vi "decodex_21.vi"() -> ()   [LabVIEW 2021]
doc: "This is a Decodex v2.1\n\nAndré Romero - 2026\nandretec@ifsc.usp.br\nIFSC - USP"
uses:
  <vilib>/Analysis/baseanly.llb/Mean (DBL).vi
  Thorlabs-Vector-Move/aptTec/Thorlabs-V2/Global Motors.vi
  <vilib>/Analysis/NI_AALBase.lvlib
panel:
  out "Layer":dbl[][](array[numeric])
  out "Motor Y":bool=TRUE
  out "Motor X":bool=TRUE
  out "Motor Z":bool=TRUE
  out "Estimated final time":string
  out "Total Estimated Time":string
  out "Total Layer Time":string
  in  "Dynamic/Manual":bool=TRUE
  in  "Mult factor":dbl=1.0
  out "Current velocity (m/s)":dbl=100.0
  out "End time":string
  out "Start time":string="5:55 PM"
  out "Total Time":string
  in  "Stop Button":bool
  out "Total Lines":i32=41
  out "Total Layers":i32=27
  out "Z initial":dbl=0.020260028541088104 format="%#_2g"
  in  "Z on/off":bool=TRUE
  in  "Layer height (mm)":dbl=1.0
  in  "file path (use dialog)":path=path "C:/user-Lab/AndreTec/SolidWorks/cubo_3_LH_06um_LW_06um_lines_3_XYSV.txt"
  out "Layer":i32=1
  out "Line":i32
  in  "Velocity (m/s)":dbl=30.0
  in  "X":refnum<k7>(container)
  in  "Y":refnum<k7>(container)
  in  "Z":refnum<k7>(container)
  # "mm"
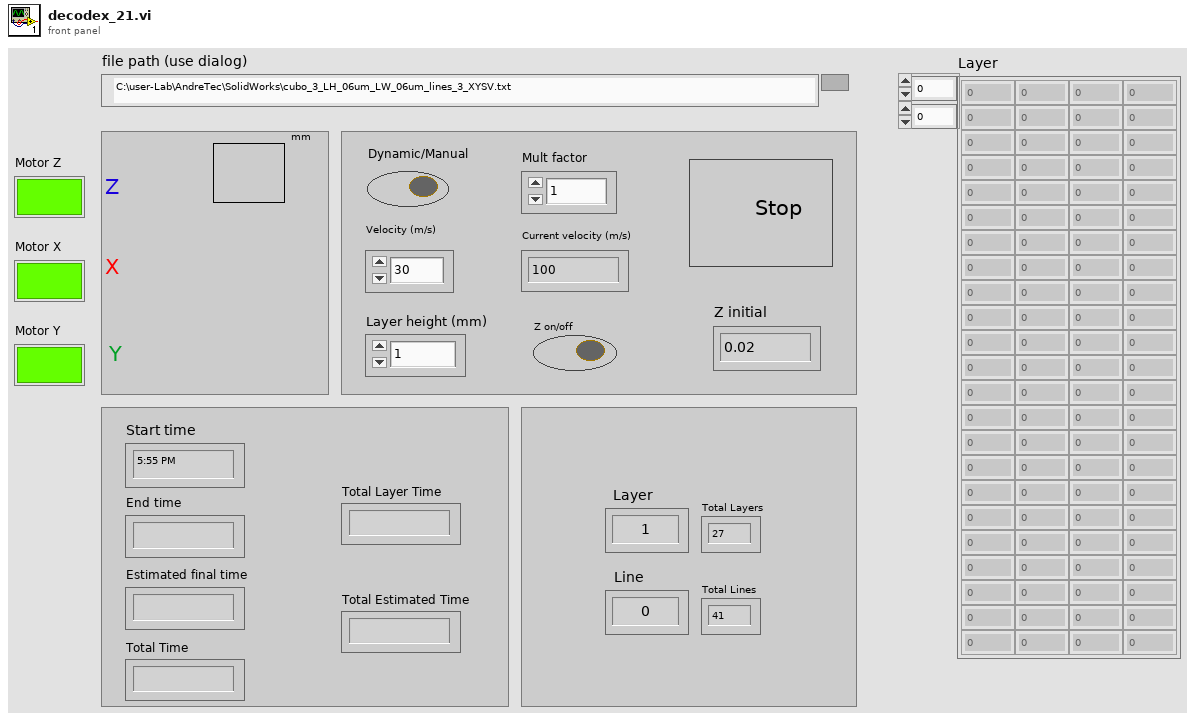
[diagram p1: front panel]
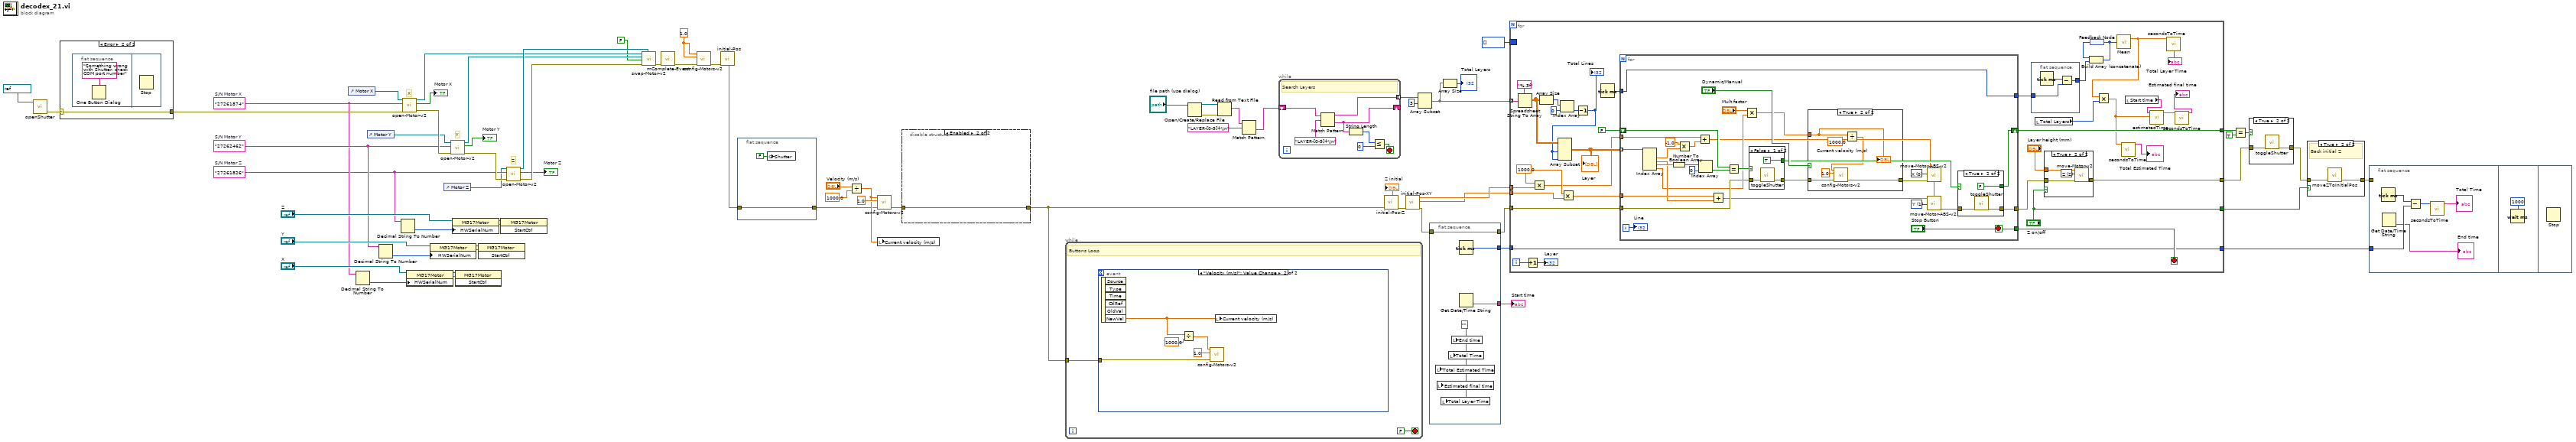
[diagram p0: block diagram]
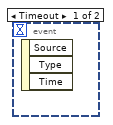
[diagram p2: hidden frame]
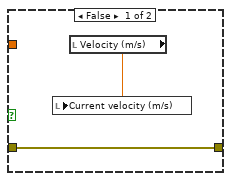
[diagram p7: hidden frame]
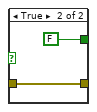
[diagram p8: hidden frame]
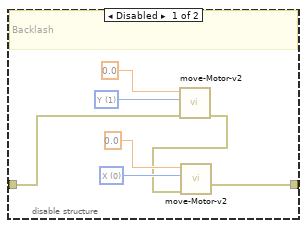
[diagram p9: hidden frame]
diagram:
  w65 = 1.0 ("Acc")
  w52 = "27262462"  # S/N Motor Y
  w51 = "27261874"  # S/N Motor X
  w42 = "27261826"  # S/N Motor Z
  # "X"
  # "Y"
  # "Z"
  n1 = call "openShutter.vi"("VISA Refnum in"=refnum<visa-resource-name> "COM3") -> ("error out"=w44:errorcluster)  [unwired: 9 in, 1 out]
  n2 = case shown="Error" w44 {
    selector: w44 -> [w71 w72]
    tunnel: [w71 w72] -> w43
    frame No Error {
    }
    frame Error {
      n3 = flat-sequence {
        frame #0 {
          n4 = One Button Dialog(message="Something wrong with Shutter, check COM port number") -> ()  [unwired: 1 in, 1 out]
        }
        frame #1 {
          n5 = Stop() -> ()  [unwired: 1 in]
        }
      }
    }
  }
  n6 = control-ref of="Motor X"() -> (w3:refnum<vi>)
  n7 = Decimal String To Number(string=w51) -> (number=w53:i32)  [unwired: 2 in, 1 out]
  n8 = control-ref of="Motor Y"() -> (w2:refnum<vi>)
  n9 = Decimal String To Number(string=w52) -> (number=w57:i32)  [unwired: 2 in, 1 out]
  n10 = Decimal String To Number(string=w42) -> (number=w61:i32)  [unwired: 2 in, 1 out]
  n11 = call "open-Motor-v2.vi"("Error In"=w43, "S/N Motor"=w51, "ref Boolean in"=w3) -> ("Error Out"=w70:errorcluster, "Motor Status"=→"Motor X":bool, "Refnum out"=w48:refnum<k7>)  [unwired: 6 in]
  n12 = property class="MG17Motor"(reference="X", "HWSerialNum"=w53) -> (reference out=w54:refnum<k7>, error out=w55:errorcluster)  [unwired: 1 in]
  n13 = property class="MG17Motor"(reference="Y", "HWSerialNum"=w57) -> (reference out=w58:refnum<k7>, error out=w59:errorcluster)  [unwired: 1 in]
  n14 = control-ref of="Motor Z"() -> (w1:refnum<vi>)
  n15 = call "open-Motor-v2.vi"("Error In"=w70, "S/N Motor"=w52, "ref Boolean in"=w2) -> ("Error Out"=w68:errorcluster, "Motor Status"=→"Motor Y":bool, "Refnum out"=w47:refnum<k7>)  [unwired: 6 in]
  n16 = property class="MG17Motor"(reference="Z", "HWSerialNum"=w61) -> (reference out=w62:refnum<k7>, error out=w63:errorcluster)  [unwired: 1 in]
  n17 = invoke class="MG17Motor" method="StartCtrl"(reference=w54, error in=w55) -> ()  [unwired: 1 in, 3 out]
  n18 = invoke class="MG17Motor" method="StartCtrl"(reference=w58, error in=w59) -> ()  [unwired: 1 in, 3 out]
  n19 = invoke class="MG17Motor" method="StartCtrl"(reference=w62, error in=w63) -> ()  [unwired: 1 in, 3 out]
  n20 = call "open-Motor-v2.vi"("Error In"=w68, "S/N Motor"=w42, "ref Boolean in"=w1) -> ("Error Out"=w67:errorcluster, "Motor Status"=→"Motor Z":bool, "Refnum out"=w66:refnum<k7>)  [unwired: 6 in]
  n21 = call "swap-Motor-v2.vi"("Refnum in M3"=w66, "error in (no error)"=w67, "Swap motor"=FALSE, "Refnum in M2"=w47, "Refnum in M1"=w48) -> ("error out"=w50:errorcluster)  [unwired: 6 in]
  n22 = call "mComplete-Event.vi"("Error In"=w50) -> ("Error Out"=w49:errorcluster)  [unwired: 10 in]
  n23 = call "config-Motors-v2.vi"("error in"=w49, "Acc"=w65, "Velocity"=w65) -> ("error out"=w69:errorcluster)  [unwired: 8 in]
  n24 = call "initial-Pos.vi"("error in (no error)"=w69) -> ("error out"=w8:errorcluster)  [unwired: 10 in]
  n25 = flat-sequence {
    tunnel: [w75] -> w9
    tunnel: w8 -> [w75]
    frame #0 {
      n26 = global write "Global Motors.vi" "Shutter"(FALSE ("Shutter")) -> ()
    }
  }
  n27 = Divide(x="Velocity (m/s)", y=1000.0) -> (x/y=w12:dbl)
  n28 = call "config-Motors-v2.vi"("error in"=w9, "Acc"=1.0, "Velocity"=w12) -> ("error out"=w39:errorcluster)  [unwired: 8 in]
  n29 = local write "Current velocity (m/s)"(w12) -> ()
  n30 = disable-structure shown="Enabled" {
    disable-tunnel: w39 -> [w78 w83]
    disable-tunnel: [w76 w83] -> w11
    frame Disabled {
      w81 = u16 1 items=["X", "Y", "Z"] ("Axis")
      w82 = u16 0 items=["X", "Y", "Z"] ("Axis")
      # "Backlash"
      n31 = call "move-Motor-v2.vi"("error in"=w78, "Axis"=w81, "Distance (um)"=0.0) -> ("error out"=w77:errorcluster)  [unwired: 8 in]
      n32 = call "move-Motor-v2.vi"("error in"=w77, "Axis"=w82, "Distance (um)"=0.0) -> ("error out"=w76:errorcluster)  [unwired: 8 in]
    }
    frame Enabled {
    }
  }
  n33 = while {
    tunnel: w11 -> [w84]
    stop <- FALSE stop-if-true
    # "Buttons Loop"
    n34 = event shown="[1] \"Velocity (m/s)\": Value Change" {
      selector: _ -> [_ _]
      dyn-events: _ -> [_ _]
      timeout: _ -> [_ _]
      tunnel: w84 -> [_ w88]
      event Timeout {
        n35 = event-data() -> ()  [unwired: 1 in, 3 out]
      }
      event "Velocity (m/s)": Value Change {
        n36 = event-data() -> ("NewVal"=w86:dbl)  [unwired: 1 in, 5 out]
        n37 = Divide(x=w86, y=1000.0) -> (x/y=w87:dbl)
        n38 = call "config-Motors-v2.vi"("error in"=w88, "Acc"=1.0, "Velocity"=w87) -> ()  [unwired: 8 in, 1 out]
        n39 = local write "Current velocity (m/s)"(w86) -> ()
      }
    }
  }
  n40 = Open/Create/Replace File(file path (use dialog)="file path (use dialog)") -> (refnum out=w37:refnum<file>, error out=w38:errorcluster)  [unwired: 5 in, 1 out]
  n41 = Read from Text File(file (use dialog)=w37, error in=w38) -> (text=w36:string)  [unwired: 2 in, 3 out]
  n42 = Match Pattern(string=w36, regular expression="LAYER-[0-9]+\\n") -> (after substring=w34:string)  [unwired: 1 in, 3 out]
  n43 = while {
    shift-right: [w94] -> _
    shift-left: w34 -> [w96]
    tunnel: [w91] -> w33 mode=indexing
    stop <- w92 stop-if-true
    # "Search Layers"
    n44 = Match Pattern(string=w96, regular expression="LAYER-[0-9]+\\n") -> (before substring=w91:string, after substring=w94:string)  [unwired: 1 in, 2 out]
    n45 = String Length(string=w94) -> (length=w95:i32)
    n46 = Less Or Equal?(x=w95, y=0) -> (x <= y?=w92:bool)
  }
  n47 = call "initial-Pos-Z.vi"("error in (no error)"=w11) -> ("error out"=w25:errorcluster, "Z position"=→"Z initial":dbl)  [unwired: 9 in]
  n48 = call "initial-Pos-XY.vi"("error in (no error)"=w25) -> ("error out"=w18:errorcluster, "Y position"=w30:dbl, "X position"=w31:dbl)  [unwired: 8 in]
  n49 = Array Subset(array=w33, index=3) -> (w27:string[])  [unwired: 1 in]
  n50 = flat-sequence {
    tunnel: w18 -> [w101]
    tunnel: [w101] -> w17
    tunnel: [w100] -> w15
    tunnel: [w99] -> w14
    frame #0 {
      w98 = "" ("End time")
      n51 = local write "Total Estimated Time"(w98) -> ()
      n52 = local write "Estimated final time"(w98) -> ()
      n53 = local write "Total Layer Time"(w98) -> ()
      n54 = local write "Total Time"(w98) -> ()
      n55 = local write "End time"(w98) -> ()
      n56 = Tick Count (ms)() -> (millisecond timer value=w100:u32)
      n57 = Get Date/Time String() -> (time string=w99:string)  [unwired: 3 in, 1 out]
    }
  }
  n58 = Array Size(array=w27) -> (size(s)=→"Total Layers":i32)
  n59 = for {
    tunnel: w27 -> [w120] mode=indexing
    tunnel: w17 -> [w137]
    tunnel: w31 -> [w125]
    tunnel: w30 -> [w126]
    tunnel: [w132] -> w20
    tunnel: ["Z on/off"] -> w28
    tunnel: [w118] -> w23
    tunnel: w15 -> [w115]
    tunnel: [w115] -> w10
    border: u32[] [] -> [_]
    i -> [w135]
    stop <- w116 stop-if-true
    w124 = 1000.0 ("x")
    n60 = Spreadsheet String To Array(format string="%.3f", spreadsheet string=w120) -> (array=w129:dbl[][])  [unwired: 2 in]
    n61 = Increment(x=w135) -> (x+1=→"Layer":i32)
    n62 = Multiply(x=w124, y=w125) -> (x*y=w123:dbl)
    n63 = Array Size(array=w129) -> (size(s)=w131:i32[])
    n64 = Index Array(array=w131, index=0) -> (element=w128:i32)
    n65 = Multiply(x=w124, y=w126) -> (x*y=w122:dbl)
    n66 = Decrement(x=w128) -> (x-1=w119:i32)
    "Total Lines" <- w119
    n67 = Array Subset(array=w129, length (row)=w119, length (col)=w119) -> (w127:dbl[][])  [unwired: 2 in]
    "Layer" <- w127
    n68 = Tick Count (ms)() -> (millisecond timer value=w114:u32)
    n69 = for {
      tunnel: w127 -> [w147] mode=indexing
      shift-right: [w151] -> w118
      shift-left: FALSE -> [w175]
      tunnel: w137 -> [w173]
      tunnel: [w152] -> w117
      tunnel: w123 -> [w168]
      tunnel: w122 -> [w167]
      tunnel: ["Stop Button"] -> w116
      tunnel: w114 -> [w149]
      tunnel: [w149] -> w113
      i -> [w170]
      stop <- "Stop Button" stop-if-true
      w171 = u16 1 items=["X", "Y", "Z"] ("Axis")
      w172 = u16 0 items=["X", "Y", "Z"] ("Axis")
      n70 = Index Array(array=w147) -> (element #1=w166:dbl, element #2=w165:dbl, element #3=w178:dbl, element #4=w158:dbl)  [unwired: 4 in]
      n71 = Number To Boolean Array(number=w178) -> (Boolean array=w177:bool[])
      n72 = Multiply(x=-1.0, y=w166) -> (x*y=w163:dbl)
      n73 = Add(x=w168, y=w163) -> (x+y=w148:dbl)
      n74 = Index Array(array=w177, index=0) -> (element=w155:bool)
      n75 = Add(x=w167, y=w165) -> (x+y=w161:dbl)
      n76 = Equal?(x=w175, y=w155) -> (x = y?=w174:bool)
      n77 = Multiply(x="Mult factor", y=w158) -> (x*y=w156:dbl)
      n78 = case shown="False" w174 {
        tunnel: w173 -> [w194 w196]
        tunnel: [w193 w196] -> w160
        tunnel: [TRUE FALSE] -> w150
        frame False {
          n79 = call "toggleShutter.vi"("Error In"=w194) -> ("error out"=w193:errorcluster)  [unwired: 9 in]
        }
        frame True {
        }
      }
      n80 = case shown="True" "Dynamic/Manual" {
        tunnel: [w185 w191] -> w154
        tunnel: w160 -> [w185 w190]
        tunnel: w156 -> [_ w186]
        frame False {
          n81 = local read "Velocity (m/s)"() -> (w184:dbl)
          n82 = local write "Current velocity (m/s)"(w184) -> ()
        }
        frame True {
          n83 = Divide(x=w186, y=1000.0) -> (x/y=w187:dbl)
          n84 = call "config-Motors-v2.vi"("error in"=w190, "Acc"=1.0, "Velocity"=w187) -> ("error out"=w191:errorcluster)  [unwired: 8 in]
          "Current velocity (m/s)" <- w186
        }
      }
      n85 = call "move-Motor-ABS-v2.vi"("error in"=w154, "Axis"=w172, "Distance (um)"=w148) -> ("error out"=w169:errorcluster)  [unwired: 8 in]
      n86 = call "move-Motor-ABS-v2.vi"("error in"=w169, "Axis"=w171, "Distance (um)"=w161) -> ("error out"=w153:errorcluster)  [unwired: 8 in]
      n87 = case shown="True" w150 {
        selector: w150 -> [w179 _]
        tunnel: w153 -> [w180 w183]
        tunnel: [w180 w182] -> w152
        tunnel: [w179 FALSE] -> w151
        frame False {
        }
        frame True {
          n88 = call "toggleShutter.vi"("Error In"=w183) -> ("error out"=w182:errorcluster)  [unwired: 9 in]
        }
      }
      "Line" <- w170
    }
    n89 = flat-sequence {
      tunnel: w113 -> [w140]
      tunnel: [w139] -> w111
      frame #0 {
        n90 = Tick Count (ms)() -> (millisecond timer value=w141:u32)
        n91 = Subtract(x=w141, y=w140) -> (x-y=w139:u32)
      }
    }
    n92 = local read "Total Layers"() -> (w107:i32)
    n93 = case shown="True" "Z on/off" {
      tunnel: "Layer height (mm)" -> [_ w145]
      tunnel: [w142 w144] -> w132
      tunnel: w117 -> [w142 w143]
      frame False {
      }
      frame True {
        w146 = u16 2 items=["X", "Y", "Z"] ("Axis")
        n94 = call "move-Motor-v2.vi"("error in"=w143, "Axis"=w146, "Distance (um)"=w145) -> ("error out"=w144:errorcluster)  [unwired: 8 in]
      }
    }
    n95 = feedback #1() -> (w110:u32[])
    n96 = Build Array (concatenate)(w110, w111) -> (w109:u32[])
    n97 = feedback-in #1(w109) -> ()
    n98 = call-poly <vilib>:"Mean.vi"("X"=w109) -> ("mean"=w105:dbl)  [unwired: 1 out]
    n99 = Multiply(x=w105, y=w107) -> (x*y=w102:dbl)
    n100 = call "secondsToTime.vi"("Time input (ms)"=w102) -> ("Time Stamp"=→"Total Estimated Time":string)  [unwired: 10 in]
    n101 = local read "Start time"() -> (w106:string)
    n102 = call "estimatedTime.vi"("time (ms)"=w102, "Start time"=w106) -> ("total time"=w104:dbl)  [unwired: 9 in]
    n103 = call "secondsToTime.vi"("Time input (ms)"=w105) -> ("Time Stamp"=→"Total Layer Time":string)  [unwired: 10 in]
    n104 = call "secondsToTime.vi"("Time input (ms)"=w104) -> ("Time Stamp"=→"Estimated final time":string)  [unwired: 10 in]
  }
  n105 = Equal?(x=w23, y=TRUE) -> (x = y?=w21:bool)
  n106 = case shown="True" w21 {
    tunnel: w20 -> [w197 w199]
    tunnel: [w197 w198] -> w19
    frame False {
    }
    frame True {
      n107 = call "toggleShutter.vi"("Error In"=w199) -> ("error out"=w198:errorcluster)  [unwired: 9 in]
    }
  }
  n108 = case shown="True" w28 {
    tunnel: [w200 w202] -> w16
    tunnel: w19 -> [w200 w201]
    frame False {
    }
    frame True {
      # "Back initial Z"
      n109 = call "moveZToInitialPos.vi"("error in"=w201) -> ("error out"=w202:errorcluster)  [unwired: 10 in]
    }
  }
  n110 = flat-sequence {
    tunnel: w16 -> [_]
    tunnel: w10 -> [w204]
    frame #0 {
      n111 = Tick Count (ms)() -> (millisecond timer value=w205:u32)
      n112 = Get Date/Time String() -> (time string=→"End time":string)  [unwired: 3 in, 1 out]
      n113 = Subtract(x=w205, y=w204) -> (x-y=w206:u32)
      n114 = call "secondsToTime.vi"("Time input (ms)"=w206) -> ("Time Stamp"=→"Total Time":string)  [unwired: 10 in]
    }
    frame #1 {
      n115 = Wait (ms)(milliseconds to wait=u32 1000) -> ()  [unwired: 1 out]
    }
    frame #2 {
      n116 = Stop() -> ()  [unwired: 1 in]
    }
  }
  "Start time" <- w14
